vi "buildTestLog.vi"(8 "error in (no error)":errorcluster, 9 "Serial Number":string, 10 "TestLogTypes":T1, 11 "TestLogFactory in":refnum<class "TestLogFactory.lvclass">) -> (0 "error out":errorcluster, 2 "ITestLog.lvclass":refnum<class "ITestLog.lvclass">, 3 "TestLogFactory out":refnum<class "TestLogFactory.lvclass">)   [LabVIEW 2016, in "TestLogFactory.lvclass"]
uses:
  TestLogFactory.lvclass
  Typedefs/TestLogTypes.ctl
  TestLog/ITestLog/ITestLog.lvclass
  Common_ConfigurationReader/ConfigurationReader.lvclass
  TestLog/CSVTestLog/CSVTestLog.lvclass
  D:/Code/ts_dcabt/Model/TestLog/ITestLog/ITestLog.lvclass
  Common_Log/Config/Log.ctl
  Common_Log/Log.lvlib
  Typedefs/ILCBTTypedefs.lvlib
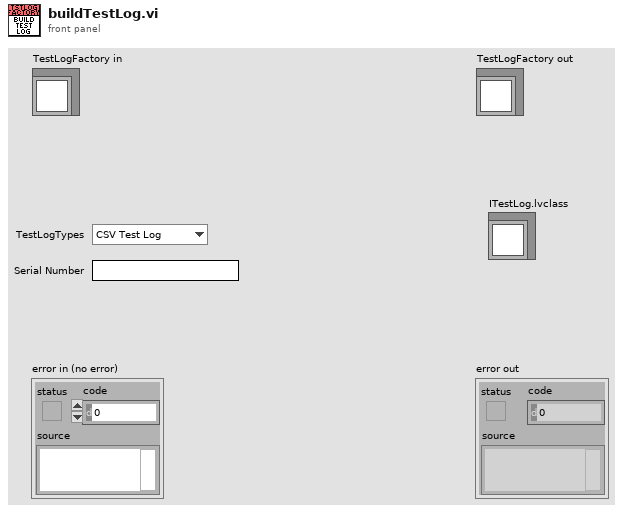
[diagram p1: front panel]
types:
  T1 = typedef "ILCBTTypedefs.lvlib/TestLogTypes.ctl" = enum16{"CSV Test Log"}
  T2 = typedef "Log.lvlib/Log.ctl" = cluster{"Log Directory":path, "Log Filename Base":string, "Max records per file":u32, "Comment":string}
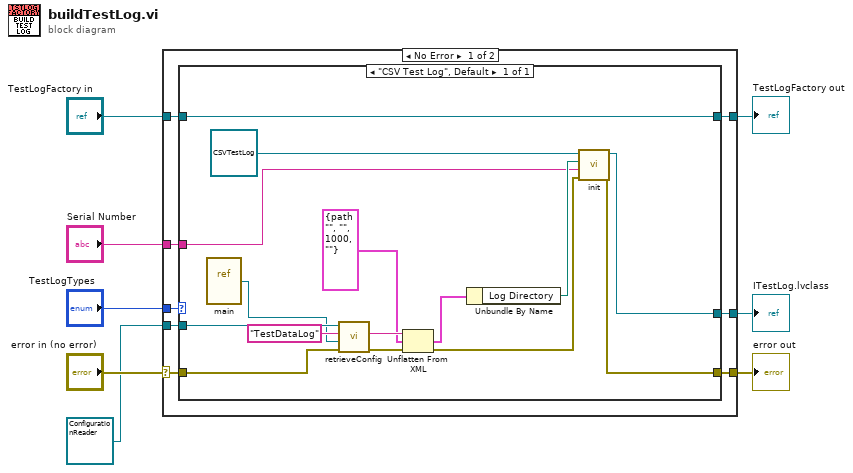
[diagram p0: block diagram]
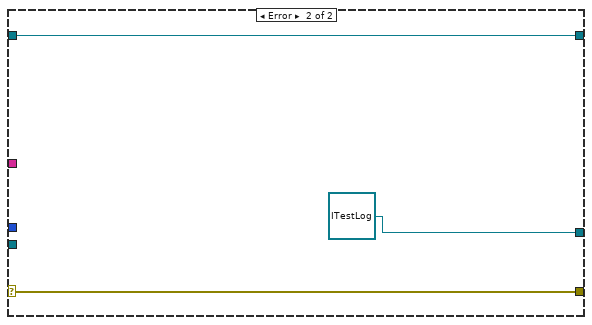
[diagram p2: hidden frame]
diagram:
  n1 = case shown="No Error" "error in (no error)" {
    selector: "error in (no error)" -> [w15 w33]
    tunnel: "TestLogTypes" -> [w16 _]
    tunnel: [w14 refnum<class "ITestLog.lvclass"> refnum ("ITestLog.lvclass")] -> w6
    tunnel: [w13 w33] -> w5
    tunnel: [w12 w34] -> w4
    tunnel: "TestLogFactory in" -> [w11 w34]
    tunnel: refnum<class "ConfigurationReader.lvclass"> refnum ("ConfigurationReader.lvclass") -> [w10 _]
    tunnel: "Serial Number" -> [w9 _]
    frame No Error {
      n2 = case shown="\"CSV Test Log\", Default" w16 {
        tunnel: w15 -> [w26]
        tunnel: [w30] -> w14
        tunnel: [w19] -> w13
        tunnel: [w31] -> w12
        tunnel: w11 -> [w31]
        tunnel: w10 -> [w28]
        tunnel: w9 -> [w18]
        frame "CSV Test Log", Default {
          n3 = vi-ref "main.vi"() -> (w17:refnum<vi>)
          n4 = call "retrieveConfig.vi"("error in (no error)"=w26, "callingVIRef"=w17, "configName"="TestDataLog", "ConfigurationReader in"=w28) -> ("error out"=w24:errorcluster, "xmlData"=w25:string)  [unwired: 5 in, 1 out]
          n5 = Unflatten From XML(xml string=w25, type=T2 {"Log Directory"=path "", "Log Filename Base"="", "Max records per file"=1000, "Comment"=""} ("Log"), error in (no error)=w24) -> (value=w22:T2, error out=w20:errorcluster)
          n6 = Unbundle By Name(w22) -> ("Log Directory"=w21:path)
          n7 = call "init.vi"("error in (no error)"=w20, "SerialNumber"=w18, "LogPath"=w21, "CSVTestLog in"=refnum<class "CSVTestLog.lvclass"> refnum ("CSVTestLog.lvclass")) -> ("error out"=w19:errorcluster, "CSVTestLog out"=w30:refnum<class "CSVTestLog.lvclass">)  [unwired: 6 in]
        }
      }
    }
    frame Error {
    }
  }
  "error out" <- w5
  "TestLogFactory out" <- w4
  "ITestLog.lvclass" <- w6
